vi "FRCts20_WebMethods_Cluster2Plain.vi"(8 "error in (no error)":errorcluster, 11 "Cluster":variant) -> (0 "error out":errorcluster, 3 "plain text":string)   [LabVIEW 2014, in "FRCts20_WebMethods.lvlib"]
doc: "Converts <B>Cluster</B> to plain text output."
uses:
  FRCts20_WebMethods.lvlib
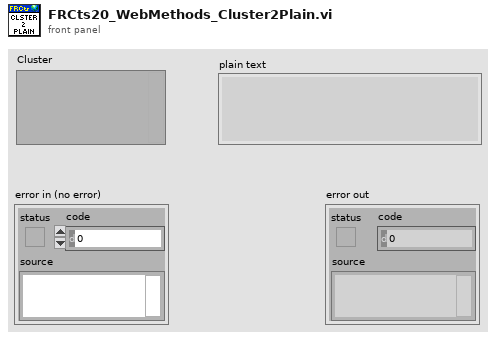
[diagram p1: front panel]
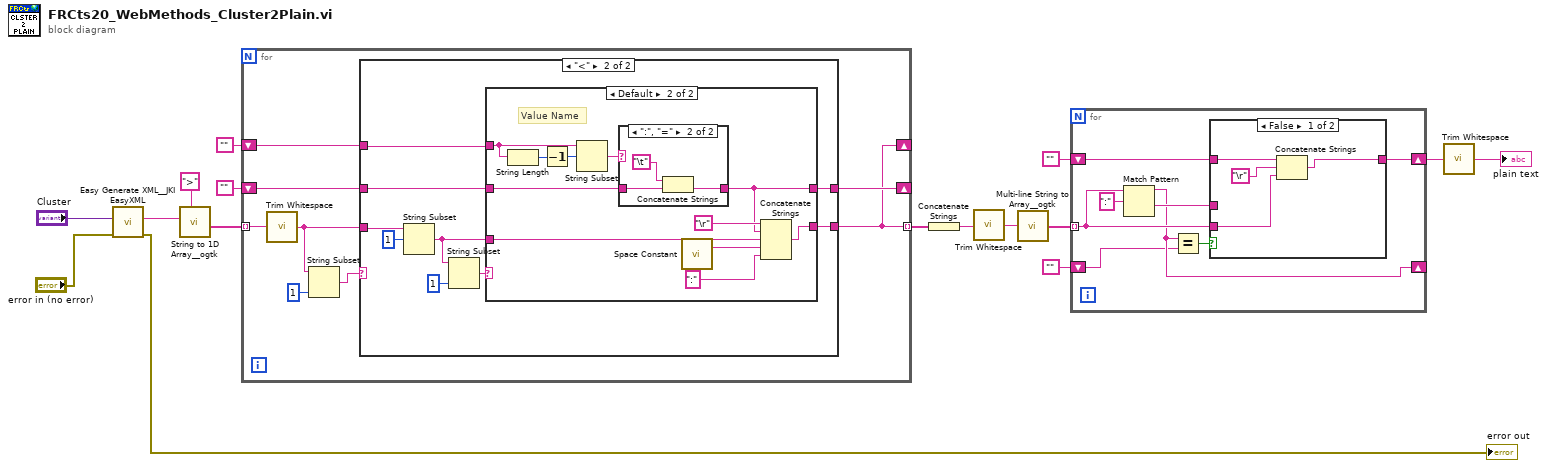
[diagram p0: block diagram]
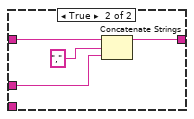
[diagram p2: hidden frame]
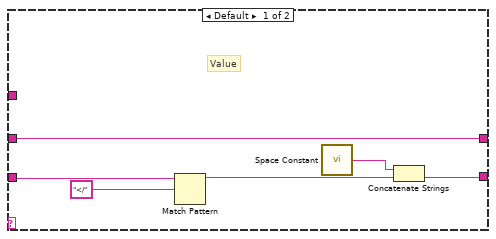
[diagram p3: hidden frame]
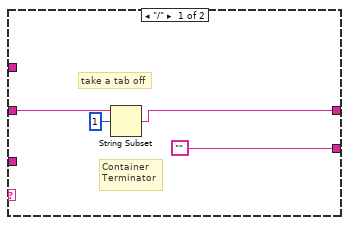
[diagram p4: hidden frame]
diagram:
  n1 = call <vilib>:"Easy Generate XML__JKI EasyXML.vi"("error in (no error)"="error in (no error)", "LabVIEW Data"="Cluster") -> ("error out"=→"error out":errorcluster, "XML String"=w4:string)  [unwired: 8 in]
  n2 = call <userlib>:"String to 1D Array__ogtk.vi"("delimiter (Tab)"=">", "string"=w4) -> ("Array of Strings"=w15:string[])  [unwired: 9 in]
  n3 = for {
    tunnel: w15 -> [w24] mode=indexing
    shift-right: [w17] -> _
    shift-left: "" -> [w20]
    shift-right: [w18] -> _
    shift-left: "" -> [w19]
    tunnel: [w17] -> w12 mode=indexing
    n4 = call <vilib>:"Trim Whitespace.vi"("string"=w24) -> ("trimmed string"=w21:string)  [unwired: 1 in]
    n5 = String Subset(string=w21, length (rest)=1 ("length (rest)")) -> (substring=w22:string)  [unwired: 1 in]
    n6 = case shown="\"<\"" w22 {
      tunnel: w21 -> [w30 w38]
      tunnel: [w26 w31] -> w17
      tunnel: w20 -> [_ w34]
      tunnel: w19 -> [w25 w33]
      tunnel: [w25 w32] -> w18
      frame Default {
        # "Value"
        n7 = Match Pattern(string=w30, regular expression="</") -> (before substring=w28:string)  [unwired: 1 in, 3 out]
        n8 = call <vilib>:"Space Constant.vi"() -> ("String"=w27:string)
        n9 = Concatenate Strings(w27, w28) -> (w26:string)
      }
      frame "<" {
        n10 = String Subset(string=w38, offset (0)=1 ("index")) -> (substring=w36:string)  [unwired: 1 in]
        n11 = String Subset(string=w36, length (rest)=1 ("length (rest)")) -> (substring=w37:string)  [unwired: 1 in]
        n12 = case shown="Default" w37 {
          tunnel: w36 -> [_ w54]
          tunnel: ["" w53] -> w31
          tunnel: w34 -> [_ w47]
          tunnel: w33 -> [w42 w46]
          tunnel: [w40 w44] -> w32
          frame "/" {
            # "take a tab off"
            # "Container\nTerminator"
            n13 = String Subset(string=w42, offset (0)=1) -> (substring=w40:string)  [unwired: 1 in]
          }
          frame Default {
            # "Value Name"
            n14 = String Length(string=w47) -> (length=w50:i32)
            n15 = Decrement(x=w50) -> (x-1=w49:i32)
            n16 = String Subset(string=w47, offset (0)=w49) -> (substring=w48:string)  [unwired: 1 in]
            n17 = case shown="\":\", \"=\"" w48 {
              tunnel: w46 -> [w55 w58]
              tunnel: [w55 w57] -> w44
              frame Default {
              }
              frame ":", "=" {
                n18 = Concatenate Strings("\t", w58) -> (w57:string)
              }
            }
            n19 = call <vilib>:"Space Constant.vi"() -> ("String"=w52:string)
            n20 = Concatenate Strings("\r", w44, w54, w52, ":") -> (w53:string)
          }
        }
      }
    }
  }
  n21 = Concatenate Strings(w12) -> (w6:string)
  n22 = call <vilib>:"Trim Whitespace.vi"("string"=w6) -> ("trimmed string"=w5:string)  [unwired: 1 in]
  n23 = call <userlib>:"Multi-line String to Array__ogtk.vi"("string"=w5) -> ("lines"=w9:string[])
  n24 = for {
    tunnel: w9 -> [w64] mode=indexing
    shift-right: [w60] -> _
    shift-left: "" -> [w59]
    shift-right: [w61] -> w8
    shift-left: "" -> [w62]
    n25 = Match Pattern(string=w64, regular expression=":") -> (before substring=w60:string, after substring=w63:string)  [unwired: 1 in, 2 out]
    n26 = Equal?(x=w60, y=w59) -> (x = y?=w65:bool)
    n27 = case shown="False" w65 {
      tunnel: w64 -> [w68 _]
      tunnel: w63 -> [_ w72]
      tunnel: w62 -> [w70 w74]
      tunnel: [w69 w71] -> w61
      frame False {
        n28 = Concatenate Strings(w70, "\r", w68) -> (w69:string)
      }
      frame True {
        n29 = Concatenate Strings(w74, "," ("string"), w72) -> (w71:string)
      }
    }
  }
  n30 = call <vilib>:"Trim Whitespace.vi"("string"=w8) -> ("trimmed string"=→"plain text":string)  [unwired: 1 in]
